vi "Sound generation.vi"(10 "sensor selector":i32, 11 "cm distance":i32) -> (3 "sine out":i16)   [LabVIEW 2014]
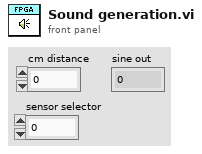
[diagram p1: front panel]
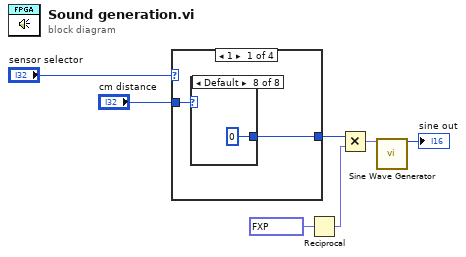
[diagram p0: block diagram]
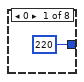
[diagram p2: hidden frame]
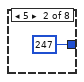
[diagram p3: hidden frame]
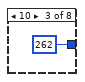
[diagram p4: hidden frame]
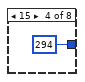
[diagram p5: hidden frame]
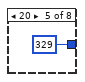
[diagram p6: hidden frame]
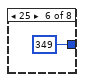
[diagram p7: hidden frame]
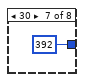
[diagram p8: hidden frame]
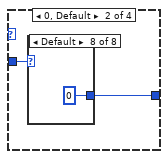
[diagram p9: hidden frame]
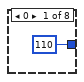
[diagram p10: hidden frame]
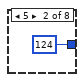
[diagram p11: hidden frame]
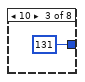
[diagram p12: hidden frame]
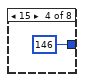
[diagram p13: hidden frame]
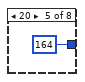
[diagram p14: hidden frame]
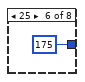
[diagram p15: hidden frame]
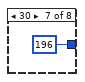
[diagram p16: hidden frame]
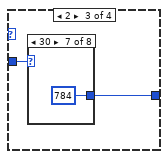
[diagram p17: hidden frame]
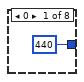
[diagram p18: hidden frame]
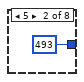
[diagram p19: hidden frame]
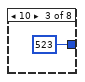
[diagram p20: hidden frame]
diagram:
  n1 = case shown="1" "sensor selector" {
    tunnel: [w8 w19 w28 w38] -> w3
    tunnel: "cm distance" -> [w9 w18 w29 w39]
    frame 1 {
      n2 = case shown="Default" w9 {
        tunnel: [220 ("frequency (periods/tick)") 247 ("frequency (periods/tick)") 262 ("frequency (periods/tick)") 294 ("frequency (periods/tick)") 329 ("frequency (periods/tick)") 349 ("frequency (periods/tick)") 392 ("frequency (periods/tick)") 0 ("frequency (periods/tick)")] -> w8
        frame 0 {
        }
        frame 5 {
        }
        frame 10 {
        }
        frame 15 {
        }
        frame 20 {
        }
        frame 25 {
        }
        frame 30 {
        }
        frame Default {
        }
      }
    }
    frame 0, Default {
      n3 = case shown="Default" w18 {
        tunnel: [110 ("frequency (periods/tick)") 124 ("frequency (periods/tick)") 131 ("frequency (periods/tick)") 146 ("frequency (periods/tick)") 164 ("frequency (periods/tick)") 175 ("frequency (periods/tick)") 196 ("frequency (periods/tick)") 0 ("frequency (periods/tick)")] -> w19
        frame 0 {
        }
        frame 5 {
        }
        frame 10 {
        }
        frame 15 {
        }
        frame 20 {
        }
        frame 25 {
        }
        frame 30 {
        }
        frame Default {
        }
      }
    }
    frame 2 {
      n4 = case shown="30" w29 {
        tunnel: [440 ("frequency (periods/tick)") 493 ("frequency (periods/tick)") 523 ("frequency (periods/tick)") 587 ("frequency (periods/tick)") 659 ("frequency (periods/tick)") 698 ("frequency (periods/tick)") 784 ("frequency (periods/tick)") 0 ("frequency (periods/tick)")] -> w28
        frame 0 {
        }
        frame 5 {
        }
        frame 10 {
        }
        frame 15 {
        }
        frame 20 {
        }
        frame 25 {
        }
        frame 30 {
        }
        frame Default {
        }
      }
    }
    frame 3 {
      n5 = case shown="30" w39 {
        tunnel: [880 ("frequency (periods/tick)") 988 ("frequency (periods/tick)") 1047 ("frequency (periods/tick)") 1175 ("frequency (periods/tick)") 1319 ("frequency (periods/tick)") 1397 ("frequency (periods/tick)") 1568 ("frequency (periods/tick)") 0 ("frequency (periods/tick)")] -> w38
        frame 0 {
        }
        frame 5 {
        }
        frame 10 {
        }
        frame 15 {
        }
        frame 20 {
        }
        frame 25 {
        }
        frame 30 {
        }
        frame Default {
        }
      }
    }
  }
  n6 = Reciprocal(x=fxp<+,17,26> 40000000.0 ("frequency (periods/tick)")) -> (1/x=w6:fxp<+,2,-24>)
  n7 = Multiply(x=w3, y=w6) -> (x*y=w7:fxp<+/-,33,7>)
  n8 = call "Sine Wave Generator"("frequency (periods/tick)"=w7) -> ("sine out"=→"sine out":i16)  [unwired: 14 in]
